vi "straingauge_4-03-2018.vi"() -> ()   [LabVIEW 2017]
uses:
  <vilib>/Analysis/baseanly.llb/Mean (DBL).vi
  <vilib>/Analysis/NI_AALBase.lvlib
  <vilib>/ptbypt/NI_PtbyPt.lvlib
panel:
  out "Smoothed Data Chart":dynamicdata(graph)
  out "CH2-Mid":dbl format="%0.8f"
  out "CH3-Right":dbl format="%0.8f"
  out "CH1-Left":dbl caption="CH1" format="%0.8f"
  in  "Sample Length":i32=100
  in  "Initialize Smoothing":bool caption="initialize"
  in  "STOP":bool
  out "Overall Mean":dbl format="%0.10f"
  out "Saving Data":bool
  out "Filename Out":path
  in  "Filename":path=path "C:/Users/mon_englab/Desktop/LabVIEW Data/Venus Body Strain Gauge Test T-MED-5565/relaxed_1.xlsx"
  in  "Enable Export":bool=TRUE caption="Enable"
  out "Waveform Chart":dynamicdata(graph)
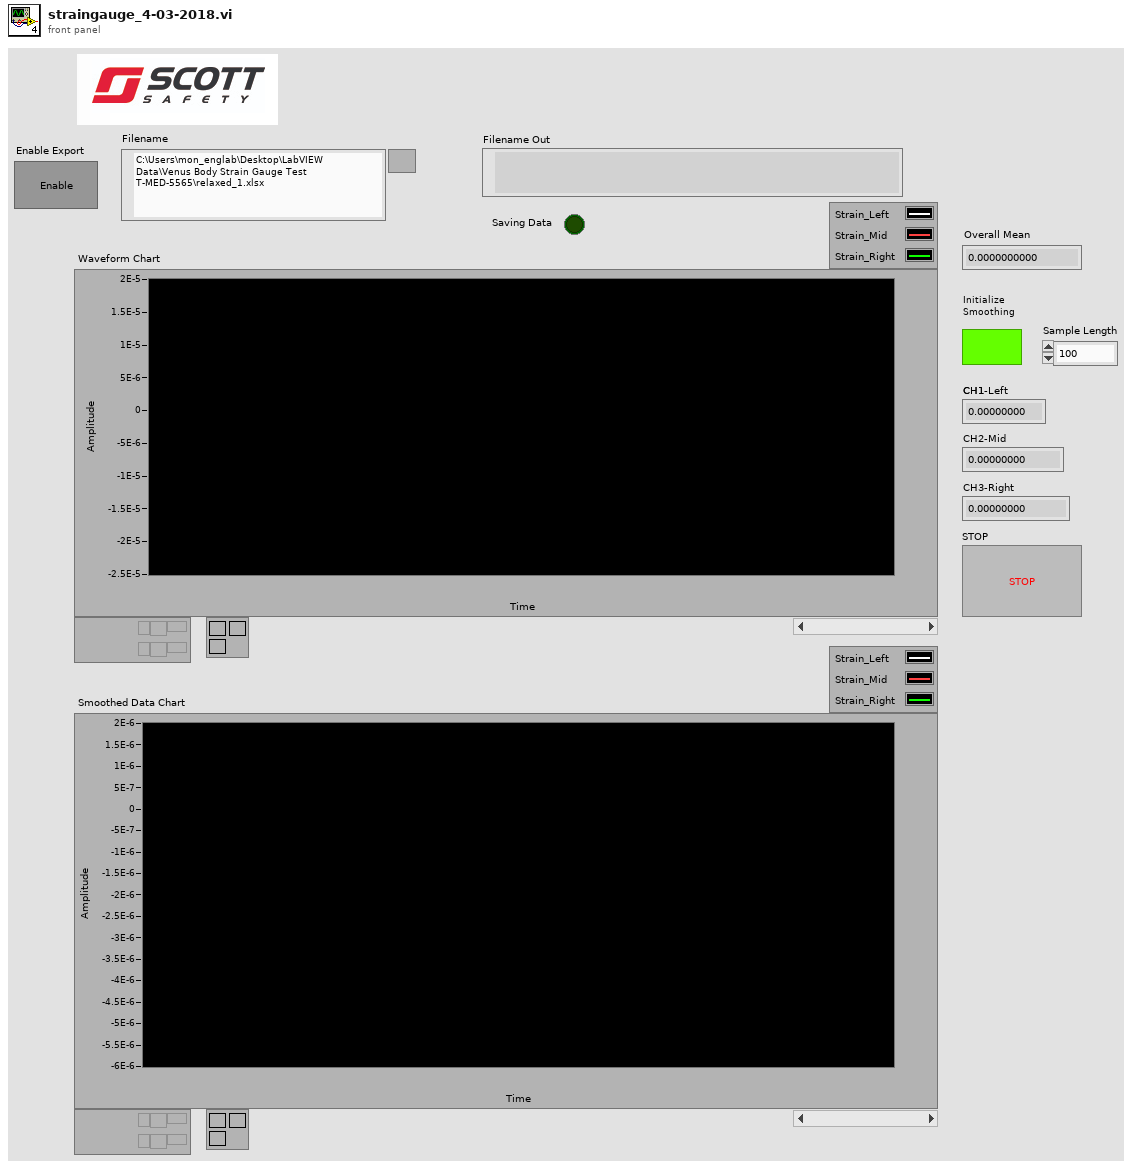
[diagram p1: front panel]
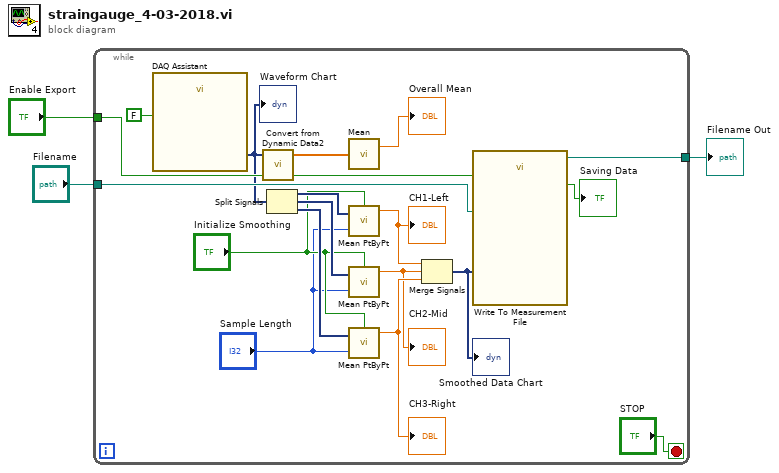
[diagram p0: block diagram]
diagram:
  n1 = while {
    tunnel: "Enable Export" -> [w14]
    tunnel: "Filename" -> [w17]
    tunnel: [w16] -> w1
    stop <- "STOP" stop-if-true
    n2 = call "DAQ Assistant"("stop (F)"=FALSE) -> ("data"=w13:dynamicdata)  [unwired: 15 in, 3 out]
    "Waveform Chart" <- w13
    n3 = call "Convert from Dynamic Data2"("Dynamic Data Type"=w13) -> ("Array"=w21:dbl[])  [unwired: 3 in]
    n4 = Split Signals(w13) -> (w12:dynamicdata, w11:dynamicdata, w10:dynamicdata)  [unwired: 3 in]
    n5 = call-poly <vilib>:"Mean.vi"("X"=w21) -> ("mean"=→"Overall Mean":dbl)  [unwired: 1 out]
    n6 = call <vilib>:"Mean PtByPt.vi"("x"=w12, "sample length"="Sample Length", "initialize"="Initialize Smoothing") -> ("mean"=w7:dbl)  [unwired: 1 in, 1 out]
    "CH1-Left" <- w7
    n7 = call <vilib>:"Mean PtByPt.vi"("x"=w11, "sample length"="Sample Length", "initialize"="Initialize Smoothing") -> ("mean"=w5:dbl)  [unwired: 1 in, 1 out]
    "CH2-Mid" <- w5
    n8 = call <vilib>:"Mean PtByPt.vi"("x"=w10, "sample length"="Sample Length", "initialize"="Initialize Smoothing") -> ("mean"=w6:dbl)  [unwired: 1 in, 1 out]
    "CH3-Right" <- w6
    n9 = Merge Signals(w7, w5, w6) -> (w4:dynamicdata)
    "Smoothed Data Chart" <- w4
    n10 = call "Write To Measurement File"("Signals"=w4, "Enable"=w14, "Filename"=w17) -> ("Filename Out"=w16:path, "Saving Data"=→"Saving Data":bool)  [unwired: 14 in, 1 out]
  }
  "Filename Out" <- w1
